vi "Begin.vi"(8 "error in":errorcluster) -> (0 "error out":errorcluster)   [LabVIEW 2015]
doc: "Called before other user functions, this VI is expected to open initial I/O refnums, load in file data, and do all program initialization. Notice that the <B>error out</B> terminal is simply used for data flow. Wiring it to other structures or subVIs ensures that this VI runs first."
uses:
  <vilib>/Rock Robotics/SystemInterfaces/DIO/FPGA_DIOPWMChannel.ctl
  <vilib>/Rock Robotics/WPI/DriverStation/WPI_DriverStationRobotMode2.ctl
  <vilib>/Rock Robotics/WPI/Joystick/WPI_JoystickDeviceEnum.ctl
  <vilib>/Rock Robotics/WPI/Solenoid/WPI_SolenoidChannel.ctl
  <vilib>/Rock Robotics/SystemInterfaces/spilib/spi_bus.ctl
  <vilib>/Rock Robotics/SystemInterfaces/DIO/FPGA_DIOChannel.ctl
  <vilib>/Rock Robotics/WPI/SafetyOutput/WPI_SafetyOutputConfigMenu.ctl
  <vilib>/Rock Robotics/WPI/RobotDrive/WPI_RobotDriveOpen2MotorWithVictor.vi
  Robot Global Data.vi
  <vilib>/Rock Robotics/Network Tables/NT Write String Array.vi
  <vilib>/Rock Robotics/WPI/MotorControl/WPI_MotorControlOpen Talon.vi
  <vilib>/Rock Robotics/WPI/Solenoid/WPI_SolenoidOpenDouble.vi
  <vilib>/Rock Robotics/WPI/Gyro/WPI_GyroXRS450_SPI_Open.vi
  <vilib>/Rock Robotics/WPI/MotorControl/WPI_MotorControlOpen Victor.vi
  <vilib>/Rock Robotics/WPI/Accelerometer/InternalAccelerometer/WPI_AccelerometerInternalOpen.vi
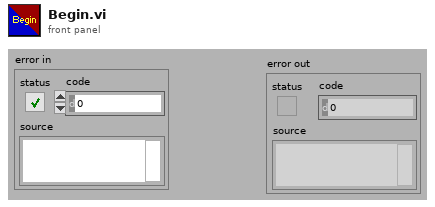
[diagram p1: front panel]
types:
  T1 = typedef "FPGA_DIOPWMChannel.ctl" = enum8{"PWM 0", "PWM 1", "PWM 2", "PWM 3", "PWM 4", "PWM 5", "PWM 6", "PWM 7", "PWM 8", "PWM 9", "PWM MXP 0", "PWM MXP 1", "PWM MXP 2", "PWM MXP 3", "PWM MXP 4", "PWM MXP 5", "PWM MXP 6", "PWM MXP 7", "PWM MXP 8", "PWM MXP 9", "Invalid"}
  T2 = typedef "WPI_SafetyOutputConfigMenu.ctl" = enum16{"Enable", "Disable"}
  T3 = typedef "WPI_JoystickDeviceEnum.ctl" = enum16{"USB 0", "USB 1", "USB 2", "USB 3", "USB 4", "USB 5"}
  T4 = typedef "FPGA_DIOChannel.ctl" = enum8{"DIO 0", "DIO 1", "DIO 2", "DIO 3", "DIO 4", "DIO 5", "DIO 6", "DIO 7", "DIO 8", "DIO 9", "DIO MXP 0", "DIO MXP 1", "DIO MXP 2", "DIO MXP 3", "DIO MXP 4", "DIO MXP 5", "DIO MXP 6", "DIO MXP 7", "DIO MXP 8", "DIO MXP 9", "DIO MXP 10", "DIO MXP 11", "DIO MXP 12", "DIO MXP 13", "DIO MXP 14", "DIO MXP 15", "Invalid"}
  T5 = typedef "WPI_SolenoidChannel.ctl" = enum8{"Solenoid 0", "Solenoid 1", "Solenoid 2", "Solenoid 3", "Solenoid 4", "Solenoid 5", "Solenoid 6", "Solenoid 7", "Invalid"}
  T6 = typedef "spi_bus.ctl" = enum16{"SPI On-Board, CS0", "SPI On-Board, CS1", "SPI On-Board, CS2", "SPI On-Board, CS3", "SPI MXP", "Invalid"}
  T7 = typedef "WPI_DriverStationRobotMode2.ctl" = enum16{"Autonomous Disabled", "Autonomous Enabled", "Teleop Disabled", "Teleop Enabled", "Disconnected", "Finish", "Test Disabled", "Test Enabled", "Emergency Stopped"}
  T8 = typedef "WPI_MotorControlDeviceRef.ctl" = cluster{"DeviceStatus":errorcluster, "Type":T9, "PWM":cluster{"PWM Channel":T1, "DeadBand":T10}, "CAN":cluster{"Device Number":u8, "Control Mode":T11, "Semaphore":T12, "Max Vout":dbl, "TalonSRX Control Mode":T13}, "Invert":bool}
  T9 = typedef "WPI_MotorControlType.ctl" = enum16{"PWM", "CAN", "CANTalonSRX"}
  T10 = typedef "WPI_PWMDeadband.ctl" = cluster{"Name":string, "maxPositivePwm":i32, "minPositivePwm":i32, "centerPwm":i32, "maxNegativePwm":i32, "minNegativePwm":i32, "angularRange":u16}
  T11 = typedef "WPI_CANJaguar_ControlMode.ctl" = enum8{"Percent VBus", "Current", "Speed", "Position", "Voltage"}
  T12 = typedef "Semaphore RefNum" = refnum<k1>
  T13 = typedef "WPI_CANTalonSRX_APIControlMode.ctl" = enum8{"Percent VBus", "Speed", "Position", "Slave", "Unchanged / Invalid", "Voltage Compensation", "Current", "Motion Profile"}
  T14 = typedef "WPI_JoystickDevRef.ctl" = cluster{"Device":T3}
  T15 = typedef "WPI_SolenoidDevRef.ctl" = cluster{"DevStatus":errorcluster, "Pneumatics Control Module":u8, "Forward Solenoid Channel":T5, "Reverse Solenoid Channel":T5}
  T16 = typedef "WPI_RobotDriveDevRef.ctl" = cluster{"DevStatus":errorcluster, "Motors[]":T8[], "Square Inputs":bool, "Max Output":dbl}
  T17 = typedef "WPI_GyroDevRef.ctl" = cluster{"DevStatus":errorcluster, "Analog Channel":T18, "Offset":dbl, "Gain (VoltsPerDegree/Second)":dbl, "Gyro Type":enum16{"Analog", "XRS450"}, "Handle":i32, "SPI Bus":T6, "Device Found":bool, "Sample Rate":dbl, "Calibrate On Open":bool}
  T18 = typedef "FPGA_AIChannel.ctl" = enum8{"AI 0", "AI 1", "AI 2", "AI 3", "AI MXP 0", "AI MXP 1", "AI MXP 2", "AI MXP 3", "Invalid"}
  T19 = typedef "WPI_ServoDeviceRef.ctl" = cluster{"DeviceStatus":errorcluster, "PWM Channel":T1, "DeadBand":T10}
  T20 = typedef "WPI_AccelerometerDevRef.ctl" = cluster{"DevStatus":errorcluster, "Scaling":T21, "Analog Channels":T22, "I2C Bus":T23, "SPI Bus":T6, "Accel Range":T24, "ADXL Axes":T25, "Handle":i32, "Device Address":u8, "Accel Type":enum16{"Analog", "ADXL345 I2C", "ADXL345 SPI", "Internal", "ADXL362 SPI"}}
  T21 = typedef "WPI_AccelerometerScaling.ctl" = cluster{"Gain (VoltsPerG)":dbl, "Center Voltage":dbl}
  T22 = typedef "WPI_AccelerometerAnalogChannels.ctl" = cluster{"X-Axis":T18, "Y-Axis":T18, "Z-Axis":T18}
  T23 = typedef "i2c_bus.ctl" = enum16{"I2C On-Board", "I2C MXP", "Invalid"}
  T24 = typedef "ADXL345 Range.ctl" = u8
  T25 = typedef "WPI_AccelerometerADXL345 Axes.ctl" = cluster{"X-Axis":bool, "Y-Axis":bool, "Z-Axis":bool}
  T26 = typedef "WPI_DigitalInputDevRef.ctl" = cluster{"DevStatus":errorcluster, "DIO Channel":T4}
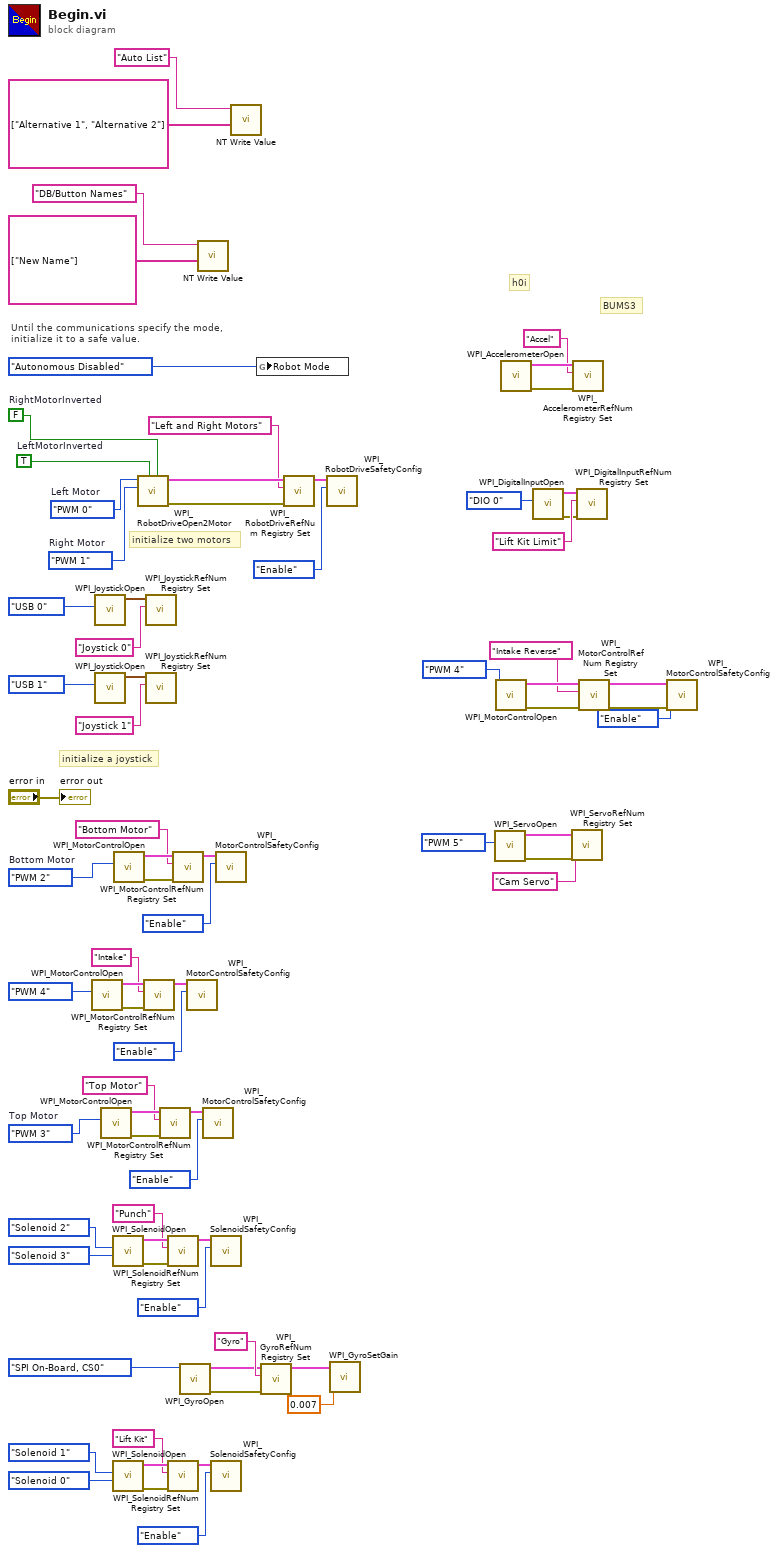
[diagram p0: block diagram]
diagram:
  w58 = FPGA_DIOPWMChannel."PWM 3"  # Top Motor
  w59 = FPGA_DIOPWMChannel."PWM 2"  # Bottom Motor
  w71 = FPGA_DIOPWMChannel."PWM 1"  # Right Motor
  w72 = FPGA_DIOPWMChannel."PWM 0"  # Left Motor
  w76 = TRUE  # LeftMotorInverted
  w77 = FALSE  # RightMotorInverted
  # "h0i"
  # "BUMS3"
  # "initialize a joystick"
  # "Until the communications specify the mode,\ninitialize it to a safe value."
  # "initialize two motors"
  n1 = call-poly <vilib>:"WPI_MotorControlOpen.vi"("PWM Channel"=FPGA_DIOPWMChannel."PWM 4") -> ("error out"=w32:errorcluster, "MotorControlDeviceRef"=w35:T8)  [unwired: 9 in]
  n2 = call <vilib>:"WPI_JoystickOpen.vi"("JoystickDevice"=WPI_JoystickDeviceEnum."USB 0") -> ("JoystickDevRef"=w66:T14)  [unwired: 10 in]
  n3 = call <vilib>:"WPI_JoystickOpen.vi"("JoystickDevice"=WPI_JoystickDeviceEnum."USB 1") -> ("JoystickDevRef"=w26:T14)  [unwired: 10 in]
  n4 = call-poly <vilib>:"WPI_MotorControlOpen.vi"("PWM Channel"=w58) -> ("error out"=w52:errorcluster, "MotorControlDeviceRef"=w57:T8)  [unwired: 9 in]
  n5 = call-poly <vilib>:"WPI_SolenoidOpen.vi"("Reverse Solenoid Channel"=WPI_SolenoidChannel."Solenoid 3", "Forward Solenoid Channel"=WPI_SolenoidChannel."Solenoid 2" ("Solenoid Channel")) -> ("error out"=w31:errorcluster, "SolenoidDevRef"=w38:T15)  [unwired: 8 in]
  n6 = call-poly <vilib>:"WPI_SolenoidOpen.vi"("Reverse Solenoid Channel"=WPI_SolenoidChannel."Solenoid 0", "Forward Solenoid Channel"=WPI_SolenoidChannel."Solenoid 1" ("Solenoid Channel")) -> ("error out"=w48:errorcluster, "SolenoidDevRef"=w51:T15)  [unwired: 8 in]
  n7 = call-poly <vilib>:"WPI_MotorControlOpen.vi"("PWM Channel"=w59) -> ("error out"=w53:errorcluster, "MotorControlDeviceRef"=w56:T8)  [unwired: 9 in]
  n8 = call-poly <vilib>:"WPI_RobotDriveOpen2Motor.vi"("Right Motor Inverted"=w77, "Left Motor Inverted"=w76, "Right Motor"=w71, "Left Motor"=w72) -> ("error out"=w73:errorcluster, "RobotDriveDevRef"=w75:T16)  [unwired: 1 in, 5 out]
  n9 = call <vilib>:"WPI_MotorControlRefNum Registry Set.vi"("error in (no error)"=w32, "refnum name"="Intake", "MotorControlDevRef"=w35) -> ("MotorControlDevRef"=w16:T8)  [unwired: 7 in, 1 out]
  n10 = call <vilib>:"WPI_JoystickRefNum Registry Set.vi"("refnum name"="Joystick 0", "JoystickDevRef"=w66) -> ()  [unwired: 8 in, 2 out]
  n11 = call <vilib>:"WPI_JoystickRefNum Registry Set.vi"("refnum name"="Joystick 1", "JoystickDevRef"=w26) -> ()  [unwired: 8 in, 2 out]
  n12 = call <vilib>:"WPI_MotorControlRefNum Registry Set.vi"("error in (no error)"=w52, "refnum name"="Top Motor", "MotorControlDevRef"=w57) -> ("MotorControlDevRef"=w24:T8)  [unwired: 7 in, 1 out]
  n13 = call <vilib>:"WPI_SolenoidRefNum Registry Set.vi"("error in (no error)"=w31, "refnum name"="Punch", "SolenoidDevRef"=w38) -> ("SolenoidDevRef"=w20:T15)  [unwired: 7 in, 1 out]
  n14 = call <vilib>:"WPI_SolenoidRefNum Registry Set.vi"("error in (no error)"=w48, "refnum name"="Lift Kit", "SolenoidDevRef"=w51) -> ("SolenoidDevRef"=w19:T15)  [unwired: 7 in, 1 out]
  n15 = call <vilib>:"WPI_MotorControlRefNum Registry Set.vi"("error in (no error)"=w53, "refnum name"="Bottom Motor", "MotorControlDevRef"=w56) -> ("MotorControlDevRef"=w23:T8)  [unwired: 7 in, 1 out]
  n16 = call-poly <vilib>:"WPI_GyroOpen.vi"("SPI Bus"=spi_bus."SPI On-Board, CS0") -> ("error out"=w42:errorcluster, "GyroDevRef"=w45:T17)  [unwired: 9 in]
  n17 = call <vilib>:"WPI_MotorControlSafetyConfig.vi"("mode"=WPI_SafetyOutputConfigMenu."Enable", "MotorControlDevRef"=w16) -> ()  [unwired: 8 in, 2 out]
  n18 = call-poly <vilib>:"NT Write Value.vi"("String Array"=string[] ["New Name"], "Name"="DB/Button Names") -> ()  [unwired: 9 in, 1 out]
  n19 = call <vilib>:"WPI_MotorControlSafetyConfig.vi"("mode"=WPI_SafetyOutputConfigMenu."Enable", "MotorControlDevRef"=w24) -> ()  [unwired: 8 in, 2 out]
  n20 = call <vilib>:"WPI_SolenoidSafetyConfig.vi"("mode"=WPI_SafetyOutputConfigMenu."Enable", "SolenoidDevRef"=w20) -> ()  [unwired: 8 in, 2 out]
  n21 = call <vilib>:"WPI_SolenoidSafetyConfig.vi"("mode"=WPI_SafetyOutputConfigMenu."Enable", "SolenoidDevRef"=w19) -> ()  [unwired: 8 in, 2 out]
  n22 = call <vilib>:"WPI_MotorControlSafetyConfig.vi"("mode"=WPI_SafetyOutputConfigMenu."Enable", "MotorControlDevRef"=w23) -> ()  [unwired: 8 in, 2 out]
  n23 = call-poly <vilib>:"NT Write Value.vi"("String Array"=string[] ["Alternative 1", "Alternative 2"], "Name"="Auto List") -> ()  [unwired: 9 in, 1 out]
  n24 = global write "Robot Global Data.vi" "Robot Mode"(WPI_DriverStationRobotMode2."Autonomous Disabled" ("Robot Mode")) -> ()
  n25 = call <vilib>:"WPI_GyroRefNum Registry Set.vi"("error in (no error)"=w42, "refnum name"="Gyro", "GyroDevRef"=w45) -> ("GyroDevRef"=w6:T17)  [unwired: 7 in, 1 out]
  n26 = call <vilib>:"WPI_RobotDriveRefNum Registry Set.vi"("error in (no error)"=w73, "refnum name"="Left and Right Motors", "RobotDriveDevRef"=w75) -> ("RobotDriveDevRef"=w70:T16)  [unwired: 1 in, 7 out]
  n27 = call <vilib>:"WPI_RobotDriveSafetyConfig.vi"("mode"=WPI_SafetyOutputConfigMenu."Enable", "RobotDriveDevRef"=w70) -> ()  [unwired: 8 in, 2 out]
  n28 = call <vilib>:"WPI_GyroSetGain.vi"("Gain (VoltsPerDegree/Second)"=0.007, "GyroDevRef"=w6) -> ()  [unwired: 8 in, 2 out]
  n29 = call <vilib>:"WPI_ServoOpen.vi"("PWM Channel"=FPGA_DIOPWMChannel."PWM 5") -> ("error out"=w1:errorcluster, "ServoDeviceRef"=w4:T19)  [unwired: 9 in]
  n30 = call-poly <vilib>:"WPI_MotorControlOpen.vi"("PWM Channel"=FPGA_DIOPWMChannel."PWM 4") -> ("error out"=w10:errorcluster, "MotorControlDeviceRef"=w13:T8)  [unwired: 9 in]
  n31 = call-poly <vilib>:"WPI_AccelerometerOpen.vi"() -> ("error out"=w40:errorcluster, "AccelerometerDevRef"=w43:T20)  [unwired: 10 in]
  n32 = call <vilib>:"WPI_DigitalInputOpen.vi"("DIO Channel"=FPGA_DIOChannel."DIO 0") -> ("error out"=w14:errorcluster, "DigitalInputDevRef"=w30:T26)  [unwired: 9 in]
  n33 = call <vilib>:"WPI_ServoRefNum Registry Set.vi"("error in (no error)"=w1, "refnum name"="Cam Servo", "ServoDeviceRef"=w4) -> ()  [unwired: 7 in, 2 out]
  n34 = call <vilib>:"WPI_AccelerometerRefNum Registry Set.vi"("error in (no error)"=w40, "refnum name"="Accel", "AccelerometerDevRef"=w43) -> ()  [unwired: 7 in, 2 out]
  n35 = call <vilib>:"WPI_DigitalInputRefNum Registry Set.vi"("error in (no error)"=w14, "refnum name"="Lift Kit Limit", "DigitalInputDevRef"=w30) -> ()  [unwired: 7 in, 2 out]
  n36 = call <vilib>:"WPI_MotorControlRefNum Registry Set.vi"("error in (no error)"=w10, "refnum name"="Intake Reverse", "MotorControlDevRef"=w13) -> ("error out"=w11:errorcluster, "MotorControlDevRef"=w12:T8)  [unwired: 7 in]
  n37 = call <vilib>:"WPI_MotorControlSafetyConfig.vi"("error in (no error)"=w11, "mode"=WPI_SafetyOutputConfigMenu."Enable", "MotorControlDevRef"=w12) -> ()  [unwired: 7 in, 2 out]
  "error out" <- "error in"
